vi "Set Strings from Ref.vi"(8 "error in (no error)":errorcluster, 9 "Language Index (0)":i32, 10 "GObj Refnum":refnum<vi>, 11 "FrontPanel in":refnum<class "FrontPanel.lvclass">) -> (0 "error out":errorcluster, 3 "FrontPanel out":refnum<class "FrontPanel.lvclass">)   [LabVIEW 2013, in "SET Project Data.lvlib" / "FrontPanel.lvclass"]
uses:
  FrontPanel.lvclass
  GObject/Read Label.vi
  GObject/GObject.lvclass
  SET Project Data.lvlib
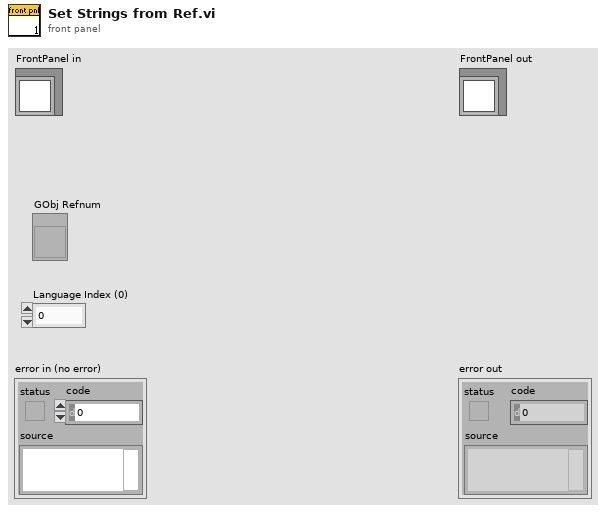
[diagram p1: front panel]
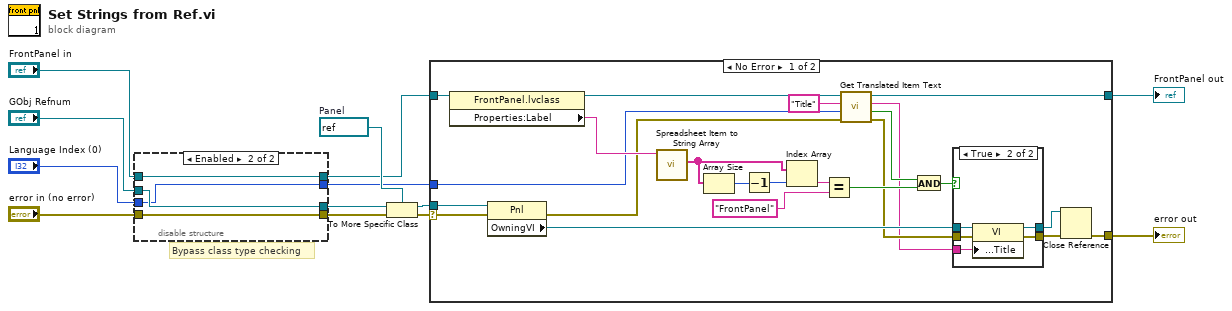
[diagram p0: block diagram]
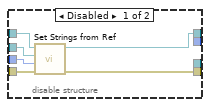
[diagram p4: hidden frame]
diagram:
  w10 = refnum<vi> refnum  # Panel
  # "Bypass class type checking"
  n1 = disable-structure shown="Enabled" {
    disable-tunnel: [w19 w22] -> w9
    disable-tunnel: [w18 w23] -> w6
    disable-tunnel: "error in (no error)" -> [w17 w22]
    disable-tunnel: "Language Index (0)" -> [w16 w20]
    disable-tunnel: "GObj Refnum" -> [w15 w21]
    disable-tunnel: "FrontPanel in" -> [w14 w23]
    disable-tunnel: [_ w21] -> w8
    disable-tunnel: [_ w20] -> w2
    frame Disabled {
      n2 = call-parent "Set Strings from Ref.vi"("error in (no error)"=w17, "Language Index (0)"=w16, "GObj Refnum"=w15, "GObject in"=w14) -> ("error out"=w19:errorcluster, "GObject out"=w18:refnum<class "FrontPanel.lvclass">)  [unwired: 6 in]
    }
    frame Enabled {
    }
  }
  n3 = To More Specific Class(target class=w10, reference=w8, error in=w9) -> (specific class reference=w3:refnum<vi>, error out=w4:errorcluster)
  n4 = case shown="No Error" w4 {
    selector: w4 -> [w35 w55]
    tunnel: w6 -> [w40 w54]
    tunnel: [w37 w54] -> w5
    tunnel: w3 -> [w36 _]
    tunnel: w2 -> [w32 _]
    tunnel: [w26 w55] -> w1
    frame No Error {
      n5 = property class="FrontPanel.lvclass"(reference=w40) -> (reference out=w38:refnum<class "FrontPanel.lvclass">, "Properties:Label"=w43:string)  [unwired: 1 in, 1 out]
      n6 = property class="Pnl"(reference=w36, error in=w35) -> (error out=w33:errorcluster, "OwningVI"=w34:refnum<vi>)  [unwired: 1 out]
      n7 = call "Spreadsheet Item to String Array.vi"("Spreadsheet Item (ASCII)"=w43) -> ("Strings [] (ASCII)"=w46:string[])  [unwired: 10 in]
      n8 = Array Size(array=w46) -> (size(s)=w44:i32)
      n9 = Decrement(x=w44) -> (x-1=w45:i32)
      n10 = Index Array(array=w46, index=w45) -> (element=w42:string)
      n11 = Equal?(x=w42, y="FrontPanel" ("element")) -> (x = y?=w31:bool)
      n12 = call "Get Translated Item Text.vi"("error in (no error)"=w33, "LangIndex (0)"=w32, "ItemName"="Title", "GObject in"=w38) -> ("error out"=w28:errorcluster, "Found?"=w30:bool, "Translated Text (ASCII)"=w24:string, "GObject out"=w37:refnum<class "FrontPanel.lvclass">)  [unwired: 4 in]
      n13 = And(x=w30, y=w31) -> (x .and. y?=w25:bool)
      n14 = case shown="True" w25 {
        tunnel: w34 -> [w48 w53]
        tunnel: [w48 w52] -> w29
        tunnel: w28 -> [w47 w51]
        tunnel: [w47 w50] -> w27
        tunnel: w24 -> [_ w49]
        frame False {
        }
        frame True {
          n15 = property class="VI"(reference=w53, error in=w51, "Front Panel.Title"=w49) -> (reference out=w52:refnum<vi>, error out=w50:errorcluster)
        }
      }
      n16 = Close Reference(reference=w29, error in (no error)=w27) -> (error out=w26:errorcluster)
    }
    frame Error {
    }
  }
  "error out" <- w1
  "FrontPanel out" <- w5
